vi "rsscope_core_global.vi"() -> ()   [LabVIEW 2014] (continued)
"Supported Models"="", "Instrument Options"="", "Flags"=0, "Help"="Return the statistic results of the specified measurement. If no parameter is specified, the result of the main measurement is returned. The main measurement is defined using RSSCOPE_ATTR_AMPT_MAIN_MEASUREMENT, RSSCOPE_ATTR_EYE_MAIN_MEASUREMENT, RSSCOPE_ATTR_HISTOGRAM_MAIN_MEASUREMENT, RSSCOPE_ATTR_JITTER_MAIN_MEASUREMENT, or RSSCOPE_ATTR_SPECTRUM_MAIN_MEASUREMENT.\n\nAvailable Repeated Capabilities:\nMeasurement: Meas1, Meas2, Meas3, Meas4, Meas5, Meas6, Meas7, Meas8, Meas9, Meas10\r\n\nRemote-control command(s):\nMEASurement<m>:RESult[:ACTual]?"}, {"Level"=3, "Class Only"=FALSE, "Identifier"="RSSCOPE_ATTR_READ_MAIN_MEASUREMENT_AVERAGE", "Descriptive Name"="Read Main Measurement Average", "Data Type"=1, "Command"="MEAS{Measurement}:RES:AVG?", "Access"=0, "Range Table"="", "Read Callback"="", "Write Callback"="", "Supported Models"="", "Instrument Options"="", "Flags"=0, "Help"="Return the statistic results of the specified measurement. If no parameter is specified, the result of the main measurement is returned. The main measurement is defined using RSSCOPE_ATTR_AMPT_MAIN_MEASUREMENT, RSSCOPE_ATTR_EYE_MAIN_MEASUREMENT, RSSCOPE_ATTR_HISTOGRAM_MAIN_MEASUREMENT, RSSCOPE_ATTR_JITTER_MAIN_MEASUREMENT, or RSSCOPE_ATTR_SPECTRUM_MAIN_MEASUREMENT.\n\nAvailable Repeated Capabilities:\nMeasurement: Meas1, Meas2, Meas3, Meas4, Meas5, Meas6, Meas7, Meas8, Meas9, Meas10\r\n\nRemote-control command(s):\nMEASurement<m>:RESult:AVG?"}, {"Level"=3, "Class Only"=FALSE, "Identifier"="RSSCOPE_ATTR_READ_MAIN_MEASUREMENT_EVENT_COUNT", "Descriptive Name"="Read Main Measurement Event Count", "Data Type"=1, "Command"="MEAS{Measurement}:RES:EVTC?", "Access"=0, "Range Table"="", "Read Callback"="", "Write Callback"="", "Supported Models"="", "Instrument Options"="", "Flags"=0, "Help"="Return the statistic results of the specified measurement. If no parameter is specified, the result of the main measurement is returned. The main measurement is defined using RSSCOPE_ATTR_AMPT_MAIN_MEASUREMENT, RSSCOPE_ATTR_EYE_MAIN_MEASUREMENT, RSSCOPE_ATTR_HISTOGRAM_MAIN_MEASUREMENT, RSSCOPE_ATTR_JITTER_MAIN_MEASUREMENT, or RSSCOPE_ATTR_SPECTRUM_MAIN_MEASUREMENT.\n\nAvailable Repeated Capabilities:\nMeasurement: Meas1, Meas2, Meas3, Meas4, Meas5, Meas6, Meas7, Meas8, Meas9, Meas10\r\n\nRemote-control command(s):\nMEASurement<m>:RESult:EVTCount?"}, {"Level"=3, "Class Only"=FALSE, "Identifier"="RSSCOPE_ATTR_READ_MAIN_MEASUREMENT_NEGATIVE_PEAK", "Descriptive Name"="Read Main Measurement Negative Peak", "Data Type"=1, "Command"="MEAS{Measurement}:RES:NPE?", "Access"=0, "Range Table"="", "Read Callback"="", "Write Callback"="", "Supported Models"="", "Instrument Options"="", "Flags"=0, "Help"="Return the statistic results of the specified measurement. If no parameter is specified, the result of the main measurement is returned. The main measurement is defined using RSSCOPE_ATTR_AMPT_MAIN_MEASUREMENT, RSSCOPE_ATTR_EYE_MAIN_MEASUREMENT, RSSCOPE_ATTR_HISTOGRAM_MAIN_MEASUREMENT, RSSCOPE_ATTR_JITTER_MAIN_MEASUREMENT, or RSSCOPE_ATTR_SPECTRUM_MAIN_MEASUREMENT.\n\nAvailable Repeated Capabilities:\nMeasurement: Meas1, Meas2, Meas3, Meas4, Meas5, Meas6, Meas7, Meas8, Meas9, Meas10\r\n\nRemote-control command(s):\nMEASurement<m>:RESult:NPEak?"}, {"Level"=3, "Class Only"=FALSE, "Identifier"="RSSCOPE_ATTR_READ_MAIN_MEASUREMENT_POSITIVE_PEAK", "Descriptive Name"="Read Main Measurement Positive Peak", "Data Type"=1, "Command"="MEAS{Measurement}:RES:PPE?", "Access"=0, "Range Table"="", "Read Callback"="", "Write Callback"="", "Supported Models"="", "Instrument Options"="", "Flags"=0, "Help"="Return the statistic results of the specified measurement. If no parameter is specified, the result of the main measurement is returned. The main measurement is defined using RSSCOPE_ATTR_AMPT_MAIN_MEASUREMENT, RSSCOPE_ATTR_EYE_MAIN_MEASUREMENT, RSSCOPE_ATTR_HISTOGRAM_MAIN_MEASUREMENT, RSSCOPE_ATTR_JITTER_MAIN_MEASUREMENT, or RSSCOPE_ATTR_SPECTRUM_MAIN_MEASUREMENT.\n\nAvailable Repeated Capabilities:\nMeasurement: Meas1, Meas2, Meas3, Meas4, Meas5, Meas6, Meas7, Meas8, Meas9, Meas10\r\n\nRemote-control command(s):\nMEASurement<m>:RESult:PPEak?"}, {"Level"=3, "Class Only"=FALSE, "Identifier"="RSSCOPE_ATTR_READ_MAIN_MEASUREMENT_RELIABILITY", "Descriptive Name"="Read Main Measurement Reliability", "Data Type"=1, "Command"="MEAS{Measurement}:RES:REL?", "Access"=0, "Range Table"="", "Read Callback"="", "Write Callback"="", "Supported Models"="", "Instrument Options"="", "Flags"=0, "Help"="Return the statistic results of the specified measurement. If no parameter is specified, the result of the main measurement is returned. The main measurement is defined using RSSCOPE_ATTR_AMPT_MAIN_MEASUREMENT, RSSCOPE_ATTR_EYE_MAIN_MEASUREMENT, RSSCOPE_ATTR_HISTOGRAM_MAIN_MEASUREMENT, RSSCOPE_ATTR_JITTER_MAIN_MEASUREMENT, or RSSCOPE_ATTR_SPECTRUM_MAIN_MEASUREMENT.\n\nAvailable Repeated Capabilities:\nMeasurement: Meas1, Meas2, Meas3, Meas4, Meas5, Meas6, Meas7, Meas8, Meas9, Meas10\r\n\nRemote-control command(s):\nMEASurement<m>:RESult:RELiability?"}, {"Level"=3, "Class Only"=FALSE, "Identifier"="RSSCOPE_ATTR_READ_MAIN_MEASUREMENT_RMS", "Descriptive Name"="Read Main Measurement RMS", "Data Type"=1, "Command"="MEAS{Measurement}:RES:RMS?", "Access"=0, "Range Table"="", "Read Callback"="", "Write Callback"="", "Supported Models"="", "Instrument Options"="", "Flags"=0, "Help"="Return the statistic results of the specified measurement. If no parameter is specified, the result of the main measurement is returned. The main measurement is defined using RSSCOPE_ATTR_AMPT_MAIN_MEASUREMENT, RSSCOPE_ATTR_EYE_MAIN_MEASUREMENT, RSSCOPE_ATTR_HISTOGRAM_MAIN_MEASUREMENT, RSSCOPE_ATTR_JITTER_MAIN_MEASUREMENT, or RSSCOPE_ATTR_SPECTRUM_MAIN_MEASUREMENT.\n\nAvailable Repeated Capabilities:\nMeasurement: Meas1, Meas2, Meas3, Meas4, Meas5, Meas6, Meas7, Meas8, Meas9, Meas10\r\n\nRemote-control command(s):\nMEASurement<m>:RESult:RMS?"}, {"Level"=3, "Class Only"=FALSE, "Identifier"="RSSCOPE_ATTR_READ_MAIN_MEASUREMENT_WAVEFORM_COUNT", "Descriptive Name"="Read Main Measurement Waveform Count", "Data Type"=1, "Command"="MEAS{Measurement}:RES:WFMC?", "Access"=0, "Range Table"="", "Read Callback"="", "Write Callback"="", "Supported Models"="", "Instrument Options"="", "Flags"=0, "Help"="Return the statistic results of the specified measurement. If no parameter is specified, the result of the main measurement is returned. The main measurement is defined using RSSCOPE_ATTR_AMPT_MAIN_MEASUREMENT, RSSCOPE_ATTR_EYE_MAIN_MEASUREMENT, RSSCOPE_ATTR_HISTOGRAM_MAIN_MEASUREMENT, RSSCOPE_ATTR_JITTER_MAIN_MEASUREMENT, or RSSCOPE_ATTR_SPECTRUM_MAIN_MEASUREMENT.\n\nAvailable Repeated Capabilities:\nMeasurement: Meas1, Meas2, Meas3, Meas4, Meas5, Meas6, Meas7, Meas8, Meas9, Meas10\r\n\nRemote-control command(s):\nMEASurement<m>:RESult:WFMCount?"}, {"Level"=3, "Class Only"=FALSE, "Identifier"="RSSCOPE_ATTR_READ_MAIN_MEASUREMENT_STANDARD_DEVIATION", "Descriptive Name"="Read Main Measurement Standard Deviation", "Data Type"=1, "Command"="MEAS{Measurement}:RES:STDD?", "Access"=0, "Range Table"="", "Read Callback"="", "Write Callback"="", "Supported Models"="", "Instrument Options"="", "Flags"=0, "Help"="Return the statistic results of the specified measurement. If no parameter is specified, the result of the main measurement is returned. The main measurement is defined using RSSCOPE_ATTR_AMPT_MAIN_MEASUREMENT, RSSCOPE_ATTR_EYE_MAIN_MEASUREMENT, RSSCOPE_ATTR_HISTOGRAM_MAIN_MEASUREMENT, RSSCOPE_ATTR_JITTER_MAIN_MEASUREMENT, or RSSCOPE_ATTR_SPECTRUM_MAIN_MEASUREMENT.\n\nAvailable Repeated Capabilities:\nMeasurement: Meas1, Meas2, Meas3, Meas4, Meas5, Meas6, Meas7, Meas8, Meas9, Meas10\r\n\nRemote-control command(s):\nMEASurement<m>:RESult:STDDev?"}, {"Level"=3, "Class Only"=FALSE, "Identifier"="RSSCOPE_ATTR_READ_REFERENCE_LEVEL_TOP_OUTER", "Descriptive Name"="Read Reference Level Top Outer", "Data Type"=1, "Command"="MEAS{Measurement}:REFL:RES:TOUT?", "Access"=0, "Range Table"="", "Read Callback"="", "Write Callback"="", "Supported Models"="", "Instrument Options"="", "Flags"=0, "Help"="Returns the area above the high signal level which is still considered to be high level.\n\nAvailable Repeated Capabilities:\nMeasurement: Meas1, Meas2, Meas3, Meas4, Meas5, Meas6, Meas7, Meas8, Meas9, Meas10\r\n\nRemote-control command(s):\nMEASurement<m>:REFLevel:RESult:TOUTer?"}, {"Level"=3, "Class Only"=FALSE, "Identifier"="RSSCOPE_ATTR_READ_REFERENCE_LEVEL_TOP_INNER", "Descriptive Name"="Read Reference Level Top Inner", "Data Type"=1, "Command"="MEAS{Measurement}:REFL:RES:TINN?", "Access"=0, "Range Table"="", "Read Callback"="", "Write Callback"="", "Supported Models"="", "Instrument Options"="", "Flags"=0, "Help"="Returns the area beneath the high signal level which is still considered to be high level.\n\nAvailable Repeated Capabilities:\nMeasurement: Meas1, Meas2, Meas3, Meas4, Meas5, Meas6, Meas7, Meas8, Meas9, Meas10\r\n\nRemote-control command(s):\nMEASurement<m>:REFLevel:RESult:TINNer?"}, {"Level"=3, "Class Only"=FALSE, "Identifier"="RSSCOPE_ATTR_READ_REFERENCE_LEVEL_BOTTOM_INNER", "Descriptive Name"="Read Reference Level Bottom Inner", "Data Type"=1, "Command"="MEAS{Measurement}:REFL:RES:BINN?", "Access"=0, "Range Table"="", "Read Callback"="", "Write Callback"="", "Supported Models"="", "Instrument Options"="", "Flags"=0, "Help"="Returns the area above the low signal level which is still considered to be low level.\n\nAvailable Repeated Capabilities:\nMeasurement: Meas1, Meas2, Meas3, Meas4, Meas5, Meas6, Meas7, Meas8, Meas9, Meas10\r\n\nRemote-control command(s):\nMEASurement<m>:REFLevel:RESult:BINNer?"}, {"Level"=3, "Class Only"=FALSE, "Identifier"="RSSCOPE_ATTR_READ_REFERENCE_LEVEL_BOTTOM_OUTER", "Descriptive Name"="Read Reference Level Bottom Outer", "Data Type"=1, "Command"="MEAS{Measurement}:REFL:RES:BOUT?", "Access"=0, "Range Table"="", "Read Callback"="", "Write Callback"="", "Supported Models"="", "Instrument Options"="", "Flags"=0, "Help"="Defines an area beneath the low signal level which is still considered to be low level.\n\nAvailable Repeated Capabilities:\nMeasurement: Meas1, Meas2, Meas3, Meas4, Meas5, Meas6, Meas7, Meas8, Meas9, Meas10\r\n\nRemote-control command(s):\nMEASurement<m>:REFLevel:RESult:BOUTer?"}, {"Level"=3, "Class Only"=FALSE, "Identifier"="RSSCOPE_ATTR_READ_REFERENCE_LEVEL_LOWER", "Descriptive Name"="Read Reference Level Lower", "Data Type"=1, "Command"="MEAS{Measurement}:REFL:RES:LOW?", "Access"=0, "Range Table"="", "Read Callback"="", "Write Callback"="", "Supported Models"="", "Instrument Options"="", "Flags"=0, "Help"="Return the lower reference level.\n\nAvailable Repeated Capabilities:\nMeasurement: Meas1, Meas2, Meas3, Meas4, Meas5, Meas6, Meas7, Meas8, Meas9, Meas10\r\n\nRemote-control command(s):\nMEASurement<m>:REFLevel:RESult:LOWer?"}, {"Level"=3, "Class Only"=FALSE, "Identifier"="RSSCOPE_ATTR_READ_REFERENCE_LEVEL_MIDDLE", "Descriptive Name"="Read Reference Level Middle", "Data Type"=1, "Command"="MEAS{Measurement}:REFL:RES:MIDD?", "Access"=0, "Range Table"="", "Read Callback"="", "Write Callback"="", "Supported Models"="", "Instrument Options"="", "Flags"=0, "Help"="Return the middle reference level.\n\nAvailable Repeated Capabilities:\nMeasurement: Meas1, Meas2, Meas3, Meas4, Meas5, Meas6, Meas7, Meas8, Meas9, Meas10\r\n\nRemote-control command(s):\nMEASurement<m>:REFLevel:RESult:MIDDle?"}, {"Level"=3, "Class Only"=FALSE, "Identifier"="RSSCOPE_ATTR_READ_REFERENCE_LEVEL_UPPER", "Descriptive Name"="Read Reference Level Upper", "Data Type"=1, "Command"="MEAS{Measurement}:REFL:RES:UPP?", "Access"=0, "Range Table"="", "Read Callback"="", "Write Callback"="", "Supported Models"="", "Instrument Options"="", "Flags"=0, "Help"="Return the upper reference level.\n\nAvailable Repeated Capabilities:\nMeasurement: Meas1, Meas2, Meas3, Meas4, Meas5, Meas6, Meas7, Meas8, Meas9, Meas10\r\n\nRemote-control command(s):\nMEASurement<m>:REFLevel:RESult:UPPer?"}, {"Level"=3, "Class Only"=FALSE, "Identifier"="RSSCOPE_ATTR_READ_REFERENCE_LEVEL_SIGNAL_LOW", "Descriptive Name"="Read Reference Level Signal Low", "Data Type"=1, "Command"="MEAS{Measurement}:REFL:RES:SIGL?", "Access"=0, "Range Table"="", "Read Callback"="", "Write Callback"="", "Supported Models"="", "Instrument Options"="", "Flags"=0, "Help"="Return the signal value that represents a low level.\n\nAvailable Repeated Capabilities:\nMeasurement: Meas1, Meas2, Meas3, Meas4, Meas5, Meas6, Meas7, Meas8, Meas9, Meas10\r\n\nRemote-control command(s):\nMEASurement<m>:REFLevel:RESult:SIGLow?"}, {"Level"=3, "Class Only"=FALSE, "Identifier"="RSSCOPE_ATTR_READ_REFERENCE_LEVEL_SIGNAL_HIGH", "Descriptive Name"="Read Reference Level Signal High", "Data Type"=1, "Command"="MEAS{Measurement}:REFL:RES:SIGH?", "Access"=0, "Range Table"="", "Read Callback"="", "Write Callback"="", "Supported Models"="", "Instrument Options"="", "Flags"=0, "Help"="Return the signal value that represents a high level.\n\nAvailable Repeated Capabilities:\nMeasurement: Meas1, Meas2, Meas3, Meas4, Meas5, Meas6, Meas7, Meas8, Meas9, Meas10\r\n\nRemote-control command(s):\nMEASurement<m>:REFLevel:RESult:SIGHigh?"}, {"Level"=3, "Class Only"=FALSE, "Identifier"="RSSCOPE_ATTR_SPECTRUM_MEASUREMENT_HARMONICS_RESULTS_NUMBER", "Descriptive Name"="Spectrum Measurement Harmonics Results Number", "Data Type"=0, "Command"="MEAS{Measurement}:RES:COUN? HAR", "Access"=0, "Range Table"="", "Read Callback"="", "Write Callback"="", "Supported Models"="", "Instrument Options"="", "Flags"=0, "Help"="Returns the number of result groups that are returned by harmonics search.\n\nAvailable Repeated Capabilities:\nMeasurement: Meas1, Meas2, Meas3, Meas4, Meas5, Meas6, Meas7, Meas8, Meas9, Meas10\r\n\nRemote-control command(s):\nMEASurement<m>:RESult:COUNt? HAR"}, {"Level"=3, "Class Only"=FALSE, "Identifier"="RSSCOPE_ATTR_DISPLAY_RESULT_LINES", "Descriptive Name"="Display Result Lines", "Data Type"=3, "Command"="MEAS{Measurement}:DISP:RES", "Access"=2, "Range Table"="", "Read Callback"="", "Write Callback"="", "Supported Models"="", "Instrument Options"="", "Flags"=0, "Help"="If enabled, the intermediate result lines required to obtain the measurement result (e.g. signal thresholds) are displayed in the measurement diagram.\n\nAvailable Repeated Capabilities:\nMeasurement: Meas1, Meas2, Meas3, Meas4, Meas5, Meas6, Meas7, Meas8, Meas9, Meas10\r\n\nRemote-control command(s):\nMEASurement<m>:DISPlay:RESults"}, {"Level"=3, "Class Only"=FALSE, "Identifier"="RSSCOPE_ATTR_DISPLAY_REFERENCE_LEVELS", "Descriptive Name"="Display Reference Levels", "Data Type"=3, "Command"="MEAS{Measurement}:DISP:LEV", "Access"=2, "Range Table"="", "Read Callback"="", "Write Callback"="", "Supported Models"="", "Instrument Options"="", "Flags"=0, "Help"="If enabled, the reference levels used for the measurement are displayed in the diagram.\n\nAvailable Repeated Capabilities:\nMeasurement: Meas1, Meas2, Meas3, Meas4, Meas5, Meas6, Meas7, Meas8, Meas9, Meas10\r\n\nRemote-control command(s):\nMEASurement<m>:DISPlay:LEVels"}, {"Level"=3, "Class Only"=FALSE, "Identifier"="RSSCOPE_ATTR_DISPLAY_RESULT_TABLE_DEFAULT_POSITION", "Descriptive Name"="Display Result Table Default Position", "Data Type"=0, "Command"="DISP:RES:MEP", "Access"=2, "Range Table"="RsScope_rngDisplayResultTableDefaultPosition", "Read Callback"="", "Write Callback"="", "Supported Models"="", "Instrument Options"="", "Flags"=0, "Help"="Defines the position of the measurement results on the display.\n\nAvailable Repeated Capabilities:\nNone\n\nRemote-control command(s):\nDISPlay:RESultboxes:MEPosition"}, {"Level"=3, "Class Only"=FALSE, "Identifier"="RSSCOPE_ATTR_DISPLAY_GROUP_RESULT_DIALOGS", "Descriptive Name"="Display Group Result Dialogs", "Data Type"=3, "Command"="MEAS:DISP:GRO", "Access"=2, "Range Table"="", "Read Callback"="", "Write Callback"="", "Supported Models"="", "Instrument Options"="", "Flags"=0, "Help"="If ON, all measurement results are shown in one result box. If disabled, the results of each measurement group are shown in a separate result box. The default position is ignored.\n\nAvailable Repeated Capabilities:\nNone\n\nRemote-control command(s):\nMEASurement<m>:DISPlay:GROuping"}, {"Level"=3, "Class Only"=TRUE, "Identifier"="", "Descriptive Name"="Raw", "Data Type"=0, "Command"="", "Access"=0, "Range Table"="", "Read Callback"="", "Write Callback"="", "Supported Models"="", "Instrument Options"="", "Flags"=0, "Help"="Use members in this class to retrieve the raw text returned by the instrument for low-level main measurements."}, {"Level"=4, "Class Only"=FALSE, "Identifier"="RSSCOPE_ATTR_READ_MAIN_MEASUREMENT_ACTUAL_STRING", "Descriptive Name"="Read Main Measurement Actual String", "Data Type"=2, "Command"="MEAS{Measurement}:RES?", "Access"=0, "Range Table"="", "Read Callback"="", "Write Callback"="", "Supported Models"="", "Instrument Options"="", "Flags"=0, "Help"="Return the statistic results of the specified measurement. If no parameter is specified, the result of the main measurement is returned. The main measurement is defined using RSSCOPE_ATTR_AMPT_MAIN_MEASUREMENT, RSSCOPE_ATTR_EYE_MAIN_MEASUREMENT, RSSCOPE_ATTR_HISTOGRAM_MAIN_MEASUREMENT, RSSCOPE_ATTR_JITTER_MAIN_MEASUREMENT, or RSSCOPE_ATTR_SPECTRUM_MAIN_MEASUREMENT.\n\nAvailable Repeated Capabilities:\nMeasurement: Meas1, Meas2, Meas3, Meas4, Meas5, Meas6, Meas7, Meas8, Meas9, Meas10\r\n\nRemote-control command(s):\nMEASurement<m>:RESult[:ACTual]?"}, {"Level"=4, "Class Only"=FALSE, "Identifier"="RSSCOPE_ATTR_READ_MAIN_MEASUREMENT_AVERAGE_STRING", "Descriptive Name"="Read Main Measurement Average String", "Data Type"=2, "Command"="MEAS{Measurement}:RES:AVG?", "Access"=0, "Range Table"="", "Read Callback"="", "Write Callback"="", "Supported Models"="", "Instrument Options"="", "Flags"=0, "Help"="Return the statistic results of the specified measurement. If no parameter is specified, the result of the main measurement is returned. The main measurement is defined using RSSCOPE_ATTR_AMPT_MAIN_MEASUREMENT, RSSCOPE_ATTR_EYE_MAIN_MEASUREMENT, RSSCOPE_ATTR_HISTOGRAM_MAIN_MEASUREMENT, RSSCOPE_ATTR_JITTER_MAIN_MEASUREMENT, or RSSCOPE_ATTR_SPECTRUM_MAIN_MEASUREMENT.\n\nAvailable Repeated Capabilities:\nMeasurement: Meas1, Meas2, Meas3, Meas4, Meas5, Meas6, Meas7, Meas8, Meas9, Meas10\r\n\nRemote-control command(s):\nMEASurement<m>:RESult:AVG?"}, {"Level"=4, "Class Only"=FALSE, "Identifier"="RSSCOPE_ATTR_READ_MAIN_MEASUREMENT_EVENT_COUNT_STRING", "Descriptive Name"="Read Main Measurement Event Count String", "Data Type"=2, "Command"="MEAS{Measurement}:RES:EVTC?", "Access"=0, "Range Table"="", "Read Callback"="", "Write Callback"="", "Supported Models"="", "Instrument Options"="", "Flags"=0, "Help"="Return the statistic results of the specified measurement. If no parameter is specified, the result of the main measurement is returned. The main measurement is defined using RSSCOPE_ATTR_AMPT_MAIN_MEASUREMENT, RSSCOPE_ATTR_EYE_MAIN_MEASUREMENT, RSSCOPE_ATTR_HISTOGRAM_MAIN_MEASUREMENT, RSSCOPE_ATTR_JITTER_MAIN_MEASUREMENT, or RSSCOPE_ATTR_SPECTRUM_MAIN_MEASUREMENT.\n\nAvailable Repeated Capabilities:\nMeasurement: Meas1, Meas2, Meas3, Meas4, Meas5, Meas6, Meas7, Meas8, Meas9, Meas10\r\n\nRemote-control command(s):\nMEASurement<m>:RESult:EVTCount?"}, {"Level"=4, "Class Only"=FALSE, "Identifier"="RSSCOPE_ATTR_READ_MAIN_MEASUREMENT_NEGATIVE_PEAK_STRING", "Descriptive Name"="Read Main Measurement Negative Peak String", "Data Type"=2, "Command"="MEAS{Measurement}:RES:NPE?", "Access"=0, "Range Table"="", "Read Callback"="", "Write Callback"="", "Supported Models"="", "Instrument Options"="", "Flags"=0, "Help"="Return the statistic results of the specified measurement. If no parameter is specified, the result of the main measurement is returned. The main measurement is defined using RSSCOPE_ATTR_AMPT_MAIN_MEASUREMENT, RSSCOPE_ATTR_EYE_MAIN_MEASUREMENT, RSSCOPE_ATTR_HISTOGRAM_MAIN_MEASUREMENT, RSSCOPE_ATTR_JITTER_MAIN_MEASUREMENT, or RSSCOPE_ATTR_SPECTRUM_MAIN_MEASUREMENT.\n\nAvailable Repeated Capabilities:\nMeasurement: Meas1, Meas2, Meas3, Meas4, Meas5, Meas6, Meas7, Meas8, Meas9, Meas10\r\n\nRemote-control command(s):\nMEASurement<m>:RESult:NPEak?"}, {"Level"=4, "Class Only"=FALSE, "Identifier"="RSSCOPE_ATTR_READ_MAIN_MEASUREMENT_POSITIVE_PEAK_STRING", "Descriptive Name"="Read Main Measurement Positive Peak String", "Data Type"=2, "Command"="MEAS{Measurement}:RES:PPE?", "Access"=0, "Range Table"="", "Read Callback"="", "Write Callback"="", "Supported Models"="", "Instrument Options"="", "Flags"=0, "Help"="Return the statistic results of the specified measurement. If no parameter is specified, the result of the main measurement is returned. The main measurement is defined using RSSCOPE_ATTR_AMPT_MAIN_MEASUREMENT, RSSCOPE_ATTR_EYE_MAIN_MEASUREMENT, RSSCOPE_ATTR_HISTOGRAM_MAIN_MEASUREMENT, RSSCOPE_ATTR_JITTER_MAIN_MEASUREMENT, or RSSCOPE_ATTR_SPECTRUM_MAIN_MEASUREMENT.\n\nAvailable Repeated Capabilities:\nMeasurement: Meas1, Meas2, Meas3, Meas4, Meas5, Meas6, Meas7, Meas8, Meas9, Meas10\r\n\nRemote-control command(s):\nMEASurement<m>:RESult:PPEak?"}, {"Level"=4, "Class Only"=FALSE, "Identifier"="RSSCOPE_ATTR_READ_MAIN_MEASUREMENT_RELIABILITY_STRING", "Descriptive Name"="Read Main Measurement Reliability String", "Data Type"=2, "Command"="MEAS{Measurement}:RES:REL?", "Access"=0, "Range Table"="", "Read Callback"="", "Write Callback"="", "Supported Models"="", "Instrument Options"="", "Flags"=0, "Help"="Return the statistic results of the specified measurement. If no parameter is specified, the result of the main measurement is returned. The main measurement is defined using RSSCOPE_ATTR_AMPT_MAIN_MEASUREMENT, RSSCOPE_ATTR_EYE_MAIN_MEASUREMENT, RSSCOPE_ATTR_HISTOGRAM_MAIN_MEASUREMENT, RSSCOPE_ATTR_JITTER_MAIN_MEASUREMENT, or RSSCOPE_ATTR_SPECTRUM_MAIN_MEASUREMENT.\n\nAvailable Repeated Capabilities:\nMeasurement: Meas1, Meas2, Meas3, Meas4, Meas5, Meas6, Meas7, Meas8, Meas9, Meas10\r\n\nRemote-control command(s):\nMEASurement<m>:RESult:RELiability?"}, {"Level"=4, "Class Only"=FALSE, "Identifier"="RSSCOPE_ATTR_READ_MAIN_MEASUREMENT_RMS_STRING", "Descriptive Name"="Read Main Measurement RMS String", "Data Type"=2, "Command"="MEAS{Measurement}:RES:RMS?", "Access"=0, "Range Table"="", "Read Callback"="", "Write Callback"="", "Supported Models"="", "Instrument Options"="", "Flags"=0, "Help"="Return the statistic results of the specified measurement. If no parameter is specified, the result of the main measurement is returned. The main measurement is defined using RSSCOPE_ATTR_AMPT_MAIN_MEASUREMENT, RSSCOPE_ATTR_EYE_MAIN_MEASUREMENT, RSSCOPE_ATTR_HISTOGRAM_MAIN_MEASUREMENT, RSSCOPE_ATTR_JITTER_MAIN_MEASUREMENT, or RSSCOPE_ATTR_SPECTRUM_MAIN_MEASUREMENT.\n\nAvailable Repeated Capabilities:\nMeasurement: Meas1, Meas2, Meas3, Meas4, Meas5, Meas6, Meas7, Meas8, Meas9, Meas10\r\n\nRemote-control command(s):\nMEASurement<m>:RESult:RMS?"}, {"Level"=4, "Class Only"=FALSE, "Identifier"="RSSCOPE_ATTR_READ_MAIN_MEASUREMENT_WAVEFORM_COUNT_STRING", "Descriptive Name"="Read Main Measurement Waveform Count String", "Data Type"=2, "Command"="MEAS{Measurement}:RES:WFMC?", "Access"=0, "Range Table"="", "Read Callback"="", "Write Callback"="", "Supported Models"="", "Instrument Options"="", "Flags"=0, "Help"="Return the statistic results of the specified measurement. If no parameter is specified, the result of the main measurement is returned. The main measurement is defined using RSSCOPE_ATTR_AMPT_MAIN_MEASUREMENT, RSSCOPE_ATTR_EYE_MAIN_MEASUREMENT, RSSCOPE_ATTR_HISTOGRAM_MAIN_MEASUREMENT, RSSCOPE_ATTR_JITTER_MAIN_MEASUREMENT, or RSSCOPE_ATTR_SPECTRUM_MAIN_MEASUREMENT.\n\nAvailable Repeated Capabilities:\nMeasurement: Meas1, Meas2, Meas3, Meas4, Meas5, Meas6, Meas7, Meas8, Meas9, Meas10\r\n\nRemote-control command(s):\nMEASurement<m>:RESult:WFMCount?"}, {"Level"=4, "Class Only"=FALSE, "Identifier"="RSSCOPE_ATTR_READ_MAIN_MEASUREMENT_STANDARD_DEVIATION_STRING", "Descriptive Name"="Read Main Measurement Standard Deviation String", "Data Type"=2, "Command"="MEAS{Measurement}:RES:STDD?", "Access"=0, "Range Table"="", "Read Callback"="", "Write Callback"="", "Supported Models"="", "Instrument Options"="", "Flags"=0, "Help"="Return the statistic results of the specified measurement. If no parameter is specified, the result of the main measurement is returned. The main measurement is defined using RSSCOPE_ATTR_AMPT_MAIN_MEASUREMENT, RSSCOPE_ATTR_EYE_MAIN_MEASUREMENT, RSSCOPE_ATTR_HISTOGRAM_MAIN_MEASUREMENT, RSSCOPE_ATTR_JITTER_MAIN_MEASUREMENT, or RSSCOPE_ATTR_SPECTRUM_MAIN_MEASUREMENT.\n\nAvailable Repeated Capabilities:\nMeasurement: Meas1, Meas2, Meas3, Meas4, Meas5, Meas6, Meas7, Meas8, Meas9, Meas10\r\n\nRemote-control command(s):\nMEASurement<m>:RESult:STDDev?"}, {"Level"=1, "Class Only"=TRUE, "Identifier"="", "Descriptive Name"="Reference Level", "Data Type"=0, "Command"="", "Access"=0, "Range Table"="", "Read Callback"="", "Write Callback"="", "Supported Models"="", "Instrument Options"="", "Flags"=0, "Help"="Contains Reference Level configuration."}, {"Level"=2, "Class Only"=FALSE, "Identifier"="RSSCOPE_ATTR_REFERENCE_LEVEL_MODE", "Descriptive Name"="Reference Level Mode", "Data Type"=0, "Command"="REFL{WfmSuffix}:LDET", "Access"=2, "Range Table"="rsscope_rngAutoManual", "Read Callback"="", "Write Callback"="", "Supported Models"="", "Instrument Options"="", "Flags"=0, "Help"="Defines whether the reference level is configured manually or automatically.\n\nAvailable Repeated Capabilities:\nWfmSuffix: WfmNone, WfmC1W1, WfmC1W2, WfmC1W3, WfmC2W1, WfmC2W2, WfmC2W3, WfmC3W1, WfmC3W2, WfmC3W3, WfmC4W1, WfmC4W2, WfmC4W3, WfmMath1, WfmMath2, WfmMath3, WfmMath4, WfmRef1, WfmRef2, WfmRef3, WfmRef4, WfmXY1, WfmXY2, WfmXY3, WfmXY4, WfmMeas1, WfmMeas2, WfmMeas3, WfmMeas4, WfmMeas5, WfmMeas6, WfmMeas7, WfmMeas8, WfmSbus1, WfmSbus2, WfmSbus3, WfmSbus4, WfmD0, WfmD1, WfmD2, WfmD3, WfmD4, WfmD5, WfmD6, WfmD7, WfmD8, WfmD9, WfmD10, WfmD11, WfmD12, WfmD13, WfmD14, WfmD15, WfmMSO1, WfmMSO2, WfmMSO3, WfmMSO4, WfmTRK1, WfmTRK2, WfmTRK3, WfmTRK4, WfmTRK5, WfmTRK6, WfmTRK7, WfmTRK8, WfmSpectrum1, WfmSpectrum2, WfmSpectrum3, WfmSpectrum4, WfmSG1TL1, WfmSG1TL2, WfmSG2TL1, WfmSG2TL2, WfmSG3TL1, WfmSG3TL2, WfmSG4TL1, WfmSG4TL2, WfmEye1, WfmEye2, WfmEye3, WfmEye4, WfmZ1V1, WfmZ1V2, WfmZ1V3, WfmZ1V4, WfmZ1I1, WfmZ1I2, WfmZ1I3, WfmZ1I4, WfmZ2V1, WfmZ2V2, WfmZ2V3, WfmZ2V4, WfmZ2I1, WfmZ2I2, WfmZ2I3, WfmZ2I4, WfmDiff1, WfmDiff2, WfmCommon1, WfmCommon2, WfmTDRZ, WfmTDRH, WfmTDRR, WfmMath5, WfmMath6, WfmMath7, WfmMath8, WfmSpectrum5, WfmSpectrum6, WfmSpectrum7, WfmSpectrum8, WfmSG5TL1, WfmSG5TL2, WfmSG6TL1, WfmSG6TL2, WfmSG7TL1, WfmSG7TL2, WfmSG8TL1, WfmSG8TL2, WfmHP1, WfmHP2, WfmHP3, WfmHP4, WfmHP5, WfmHP6, WfmHP7, WfmHP8, WfmHP9, WfmHP10, WfmBathtub1, WfmBathMeas1, WfmStepResp1, WfmSRHist1, WfmSDHist1, WfmTJHist1, WfmDJHist1, WfmDDJHist1, WfmPJHist1, WfmRJOHist1, WfmSRTrack1, WfmTJTrack1, WfmDJTrack1, WfmDDJTrack1, WfmPJTrack1, WfmRJTrack1, WfmTJSpectrum1, WfmDDJSpectrum1, WfmPJSpectrum1, WfmRJSpectrum1, WfmSEye1, WfmBathtub2, WfmBathMeas2, WfmStepResp2, WfmSRHist2, WfmSDHist2, WfmTJHist2, WfmDJHist2, WfmDDJHist2, WfmPJHist2, WfmRJOHist2, WfmSRTrack2, WfmSDTrack2, WfmTJTrack2, WfmDDJTrack2, WfmPJTrack2, WfmRJTrack2, WfmTJSpectrum2, WfmDDJSpectrum2, WfmPJSpectrum2, WfmRJSpectrum2, WfmSEye2, WfmNBathtub1, WfmNBathMeas1, WfmTNHist1, WfmDNHist1, WfmDDNHist1, WfmPNHist1, WfmRNOTrack1, WfmTNTrack1, WfmDDNTrack1, WfmPNTrack1, WfmRNTrack1, WfmTNSpectrum1, WfmDDNSpectrum1, WfmPNSpectrum1, WfmRNSpectrum1, WfmNBathtub2, WfmNBathMeas2, WfmTNHist2, WfmDNHist2, WfmDDNHist2, WfmPNHist2, WfmRNOHist2, WfmTNTrack2, WfmDDNTrack2, WfmPNTrack2, WfmRNTrack2, WfmTNSpectrum2, WfmDDNSpectrum2, WfmPNSpectrum2, WfmRNSpectrum2, WfmPJDHist1, WfmBUJHist1, WfmRJHist1, WfmPJDTrack1, WfmPJDSpectrum1, WfmPJDHist2, WfmBUJHist2, WfmRJHist2, WfmPJDTrack2, WfmPJDSpectrum2, WfmPNDHist1, WfmBUNHist1, WfmRNHist1, WfmPNDTrack1, WfmPNDSpectrum1, WfmPNDHist2, WfmBUNHist2, WfmRNHist2, WfmPNDTrack2, WfmPNDSpectrum2\r\n\nRemote-control command(s):\nREFLevel<m>:LDETection"}, {"Level"=2, "Class Only"=FALSE, "Identifier"="RSSCOPE_ATTR_REFERENCE_LEVEL_RELATIVE_LEVELS", "Descriptive Name"="Reference Level Relative Levels", "Data Type"=0, "Command"="REFL{WfmSuffix}:REL:MODE", "Access"=2, "Range Table"="rsscope_rngRefLevelRelative", "Read Callback"="", "Write Callback"="", "Supported Models"="", "Instrument Options"="", "Flags"=0, "Help"="The lower, middle and upper reference levels, defined as percentages of the high signal level.\n\nNote:\nFor user defined values set USER and use these attributes:\n\nRSSCOPE_ATTR_USER_REFERENCE_RELATIVE_LOWER_LEVEL\nRSSCOPE_ATTR_USER_REFERENCE_RELATIVE_MIDDLE_LEVEL\nRSSCOPE_ATTR_USER_REFERENCE_RELATIVE_UPPER_LEVEL\n\nAvailable Repeated Capabilities:\nWfmSuffix: WfmNone, WfmC1W1, WfmC1W2, WfmC1W3, WfmC2W1, WfmC2W2, WfmC2W3, WfmC3W1, WfmC3W2, WfmC3W3, WfmC4W1, WfmC4W2, WfmC4W3, WfmMath1, WfmMath2, WfmMath3, WfmMath4, WfmRef1, WfmRef2, WfmRef3, WfmRef4, WfmXY1, WfmXY2, WfmXY3, WfmXY4, WfmMeas1, WfmMeas2, WfmMeas3, WfmMeas4, WfmMeas5, WfmMeas6, WfmMeas7, WfmMeas8, WfmSbus1, WfmSbus2, WfmSbus3, WfmSbus4, WfmD0, WfmD1, WfmD2, WfmD3, WfmD4, WfmD5, WfmD6, WfmD7, WfmD8, WfmD9, WfmD10, WfmD11, WfmD12, WfmD13, WfmD14, WfmD15, WfmMSO1, WfmMSO2, WfmMSO3, WfmMSO4, WfmTRK1, WfmTRK2, WfmTRK3, WfmTRK4, WfmTRK5, WfmTRK6, WfmTRK7, WfmTRK8, WfmSpectrum1, WfmSpectrum2, WfmSpectrum3, WfmSpectrum4, WfmSG1TL1, WfmSG1TL2, WfmSG2TL1, WfmSG2TL2, WfmSG3TL1, WfmSG3TL2, WfmSG4TL1, WfmSG4TL2, WfmEye1, WfmEye2, WfmEye3, WfmEye4, WfmZ1V1, WfmZ1V2, WfmZ1V3, WfmZ1V4, WfmZ1I1, WfmZ1I2, WfmZ1I3, WfmZ1I4, WfmZ2V1, WfmZ2V2, WfmZ2V3, WfmZ2V4, WfmZ2I1, WfmZ2I2, WfmZ2I3, WfmZ2I4, WfmDiff1, WfmDiff2, WfmCommon1, WfmCommon2, WfmTDRZ, WfmTDRH, WfmTDRR, WfmMath5, WfmMath6, WfmMath7, WfmMath8, WfmSpectrum5, WfmSpectrum6, WfmSpectrum7, WfmSpectrum8, WfmSG5TL1, WfmSG5TL2, WfmSG6TL1, WfmSG6TL2, WfmSG7TL1, WfmSG7TL2, WfmSG8TL1, WfmSG8TL2, WfmHP1, WfmHP2, WfmHP3, WfmHP4, WfmHP5, WfmHP6, WfmHP7, WfmHP8, WfmHP9, WfmHP10, WfmBathtub1, WfmBathMeas1, WfmStepResp1, WfmSRHist1, WfmSDHist1, WfmTJHist1, WfmDJHist1, WfmDDJHist1, WfmPJHist1, WfmRJOHist1, WfmSRTrack1, WfmTJTrack1, WfmDJTrack1, WfmDDJTrack1, WfmPJTrack1, WfmRJTrack1, WfmTJSpectrum1, WfmDDJSpectrum1, WfmPJSpectrum1, WfmRJSpectrum1, WfmSEye1, WfmBathtub2, WfmBathMeas2, WfmStepResp2, WfmSRHist2, WfmSDHist2, WfmTJHist2, WfmDJHist2, WfmDDJHist2, WfmPJHist2, WfmRJOHist2, WfmSRTrack2, WfmSDTrack2, WfmTJTrack2, WfmDDJTrack2, WfmPJTrack2, WfmRJTrack2, WfmTJSpectrum2, WfmDDJSpectrum2, WfmPJSpectrum2, WfmRJSpectrum2, WfmSEye2, WfmNBathtub1, WfmNBathMeas1, WfmTNHist1, WfmDNHist1, WfmDDNHist1, WfmPNHist1, WfmRNOTrack1, WfmTNTrack1, WfmDDNTrack1, WfmPNTrack1, WfmRNTrack1, WfmTNSpectrum1, WfmDDNSpectrum1, WfmPNSpectrum1, WfmRNSpectrum1, WfmNBathtub2, WfmNBathMeas2, WfmTNHist2, WfmDNHist2, WfmDDNHist2, WfmPNHist2, WfmRNOHist2, WfmTNTrack2, WfmDDNTrack2, WfmPNTrack2, WfmRNTrack2, WfmTNSpectrum2, WfmDDNSpectrum2, WfmPNSpectrum2, WfmRNSpectrum2, WfmPJDHist1, WfmBUJHist1, WfmRJHist1, WfmPJDTrack1, WfmPJDSpectrum1, WfmPJDHist2, WfmBUJHist2, WfmRJHist2, WfmPJDTrack2, WfmPJDSpectrum2, WfmPNDHist1, WfmBUNHist1, WfmRNHist1, WfmPNDTrack1, WfmPNDSpectrum1, WfmPNDHist2, WfmBUNHist2, WfmRNHist2, WfmPNDTrack2, WfmPNDSpectrum2\r\n\nRemote-control command(s):\nREFLevel<m>:RELative:MODE"}, {"Level"=2, "Class Only"=FALSE, "Identifier"="RSSCOPE_ATTR_REFERENCE_LEVEL_USER_LEVEL", "Descriptive Name"="Reference Level User Level", "Data Type"=0, "Command"="REFL{WfmSuffix}:USRL", "Access"=2, "Range Table"="rsscope_rngUserLevel", "Read Callback"="", "Write Callback"="", "Supported Models"="", "Instrument Options"="", "Flags"=0, "Help"="Defines whether the user-defined signal levels or user-defined reference levels are used for the measurements.\n\nAvailable Repeated Capabilities:\nWfmSuffix: WfmNone, WfmC1W1, WfmC1W2, WfmC1W3, WfmC2W1, WfmC2W2, WfmC2W3, WfmC3W1, WfmC3W2, WfmC3W3, WfmC4W1, WfmC4W2, WfmC4W3, WfmMath1, WfmMath2, WfmMath3, WfmMath4, WfmRef1, WfmRef2, WfmRef3, WfmRef4, WfmXY1, WfmXY2, WfmXY3, WfmXY4, WfmMeas1, WfmMeas2, WfmMeas3, WfmMeas4, WfmMeas5, WfmMeas6, WfmMeas7, WfmMeas8, WfmSbus1, WfmSbus2, WfmSbus3, WfmSbus4, WfmD0, WfmD1, WfmD2, WfmD3, WfmD4, WfmD5, WfmD6, WfmD7, WfmD8, WfmD9, WfmD10, WfmD11, WfmD12, WfmD13, WfmD14, WfmD15, WfmMSO1, WfmMSO2, WfmMSO3, WfmMSO4, WfmTRK1, WfmTRK2, WfmTRK3, WfmTRK4, WfmTRK5, WfmTRK6, WfmTRK7, WfmTRK8, WfmSpectrum1, WfmSpectrum2, WfmSpectrum3, WfmSpectrum4, WfmSG1TL1, WfmSG1TL2, WfmSG2TL1, WfmSG2TL2, WfmSG3TL1, WfmSG3TL2, WfmSG4TL1, WfmSG4TL2, WfmEye1, WfmEye2, WfmEye3, WfmEye4, WfmZ1V1, WfmZ1V2, WfmZ1V3, WfmZ1V4, WfmZ1I1, WfmZ1I2, WfmZ1I3, WfmZ1I4, WfmZ2V1, WfmZ2V2, WfmZ2V3, WfmZ2V4, WfmZ2I1, WfmZ2I2, WfmZ2I3, WfmZ2I4, WfmDiff1, WfmDiff2, WfmCommon1, WfmCommon2, WfmTDRZ, WfmTDRH, WfmTDRR, WfmMath5, WfmMath6, WfmMath7, WfmMath8, WfmSpectrum5, WfmSpectrum6, WfmSpectrum7, WfmSpectrum8, WfmSG5TL1, WfmSG5TL2, WfmSG6TL1, WfmSG6TL2, WfmSG7TL1, WfmSG7TL2, WfmSG8TL1, WfmSG8TL2, WfmHP1, WfmHP2, WfmHP3, WfmHP4, WfmHP5, WfmHP6, WfmHP7, WfmHP8, WfmHP9, WfmHP10, WfmBathtub1, WfmBathMeas1, WfmStepResp1, WfmSRHist1, WfmSDHist1, WfmTJHist1, WfmDJHist1, WfmDDJHist1, WfmPJHist1, WfmRJOHist1, WfmSRTrack1, WfmTJTrack1, WfmDJTrack1, WfmDDJTrack1, WfmPJTrack1, WfmRJTrack1, WfmTJSpectrum1, WfmDDJSpectrum1, WfmPJSpectrum1, WfmRJSpectrum1, WfmSEye1, WfmBathtub2, WfmBathMeas2, WfmStepResp2, WfmSRHist2, WfmSDHist2, WfmTJHist2, WfmDJHist2, WfmDDJHist2, WfmPJHist2, WfmRJOHist2, WfmSRTrack2, WfmSDTrack2, WfmTJTrack2, WfmDDJTrack2, WfmPJTrack2, WfmRJTrack2, WfmTJSpectrum2, WfmDDJSpectrum2, WfmPJSpectrum2, WfmRJSpectrum2, WfmSEye2, WfmNBathtub1, WfmNBathMeas1, WfmTNHist1, WfmDNHist1, WfmDDNHist1, WfmPNHist1, WfmRNOTrack1, WfmTNTrack1, WfmDDNTrack1, WfmPNTrack1, WfmRNTrack1, WfmTNSpectrum1, WfmDDNSpectrum1, WfmPNSpectrum1, WfmRNSpectrum1, WfmNBathtub2, WfmNBathMeas2, WfmTNHist2, WfmDNHist2, WfmDDNHist2, WfmPNHist2, WfmRNOHist2, WfmTNTrack2, WfmDDNTrack2, WfmPNTrack2, WfmRNTrack2, WfmTNSpectrum2, WfmDDNSpectrum2, WfmPNSpectrum2, WfmRNSpectrum2, WfmPJDHist1, WfmBUJHist1, WfmRJHist1, WfmPJDTrack1, WfmPJDSpectrum1, WfmPJDHist2, WfmBUJHist2, WfmRJHist2, WfmPJDTrack2, WfmPJDSpectrum2, WfmPNDHist1, WfmBUNHist1, WfmRNHist1, WfmPNDTrack1, WfmPNDSpectrum1, WfmPNDHist2, WfmBUNHist2, WfmRNHist2, WfmPNDTrack2, WfmPNDSpectrum2\r\n\nRemote-control command(s):\nREFLevel<m>:USRLevel"}, {"Level"=2, "Class Only"=FALSE, "Identifier"="RSSCOPE_ATTR_REFERENCE_LEVEL_DEFINITION", "Descriptive Name"="Reference Level Definition", "Data Type"=0, "Command"="REFL{WfmSuffix}:LMOD", "Access"=2, "Range Table"="rsscope_rngAbsRel", "Read Callback"="", "Write Callback"="", "Supported Models"="", "Instrument Options"="", "Flags"=0, "Help"="Defines whether the reference is configured using absolute or relative values.\n\nAvailable Repeated Capabilities:\nWfmSuffix: WfmNone, WfmC1W1, WfmC1W2, WfmC1W3, WfmC2W1, WfmC2W2, WfmC2W3, WfmC3W1, WfmC3W2, WfmC3W3, WfmC4W1, WfmC4W2, WfmC4W3, WfmMath1, WfmMath2, WfmMath3, WfmMath4, WfmRef1, WfmRef2, WfmRef3, WfmRef4, WfmXY1, WfmXY2, WfmXY3, WfmXY4, WfmMeas1, WfmMeas2, WfmMeas3, WfmMeas4, WfmMeas5, WfmMeas6, WfmMeas7, WfmMeas8, WfmSbus1, WfmSbus2, WfmSbus3, WfmSbus4, WfmD0, WfmD1, WfmD2, WfmD3, WfmD4, WfmD5, WfmD6, WfmD7, WfmD8, WfmD9, WfmD10, WfmD11, WfmD12, WfmD13, WfmD14, WfmD15, WfmMSO1, WfmMSO2, WfmMSO3, WfmMSO4, WfmTRK1, WfmTRK2, WfmTRK3, WfmTRK4, WfmTRK5, WfmTRK6, WfmTRK7, WfmTRK8, WfmSpectrum1, WfmSpectrum2, WfmSpectrum3, WfmSpectrum4, WfmSG1TL1, WfmSG1TL2, WfmSG2TL1, WfmSG2TL2, WfmSG3TL1, WfmSG3TL2, WfmSG4TL1, WfmSG4TL2, WfmEye1, WfmEye2, WfmEye3, WfmEye4, WfmZ1V1, WfmZ1V2, WfmZ1V3, WfmZ1V4, WfmZ1I1, WfmZ1I2, WfmZ1I3, WfmZ1I4, WfmZ2V1, WfmZ2V2, WfmZ2V3, WfmZ2V4, WfmZ2I1, WfmZ2I2, WfmZ2I3, WfmZ2I4, WfmDiff1, WfmDiff2, WfmCommon1, WfmCommon2, WfmTDRZ, WfmTDRH, WfmTDRR, WfmMath5, WfmMath6, WfmMath7, WfmMath8, WfmSpectrum5, WfmSpectrum6, WfmSpectrum7, WfmSpectrum8, WfmSG5TL1, WfmSG5TL2, WfmSG6TL1, WfmSG6TL2, WfmSG7TL1, WfmSG7TL2, WfmSG8TL1, WfmSG8TL2, WfmHP1, WfmHP2, WfmHP3, WfmHP4, WfmHP5, WfmHP6, WfmHP7, WfmHP8, WfmHP9, WfmHP10, WfmBathtub1, WfmBathMeas1, WfmStepResp1, WfmSRHist1, WfmSDHist1, WfmTJHist1, WfmDJHist1, WfmDDJHist1, WfmPJHist1, WfmRJOHist1, WfmSRTrack1, WfmTJTrack1, WfmDJTrack1, WfmDDJTrack1, WfmPJTrack1, WfmRJTrack1, WfmTJSpectrum1, WfmDDJSpectrum1, WfmPJSpectrum1, WfmRJSpectrum1, WfmSEye1, WfmBathtub2, WfmBathMeas2, WfmStepResp2, WfmSRHist2, WfmSDHist2, WfmTJHist2, WfmDJHist2, WfmDDJHist2, WfmPJHist2, WfmRJOHist2, WfmSRTrack2, WfmSDTrack2, WfmTJTrack2, WfmDDJTrack2, WfmPJTrack2, WfmRJTrack2, WfmTJSpectrum2, WfmDDJSpectrum2, WfmPJSpectrum2, WfmRJSpectrum2, WfmSEye2, WfmNBathtub1, WfmNBathMeas1, WfmTNHist1, WfmDNHist1, WfmDDNHist1, WfmPNHist1, WfmRNOTrack1, WfmTNTrack1, WfmDDNTrack1, WfmPNTrack1, WfmRNTrack1, WfmTNSpectrum1, WfmDDNSpectrum1, WfmPNSpectrum1, WfmRNSpectrum1, WfmNBathtub2, WfmNBathMeas2, WfmTNHist2, WfmDNHist2, WfmDDNHist2, WfmPNHist2, WfmRNOHist2, WfmTNTrack2, WfmDDNTrack2, WfmPNTrack2, WfmRNTrack2, WfmTNSpectrum2, WfmDDNSpectrum2, WfmPNSpectrum2, WfmRNSpectrum2, WfmPJDHist1, WfmBUJHist1, WfmRJHist1, WfmPJDTrack1, WfmPJDSpectrum1, WfmPJDHist2, WfmBUJHist2, WfmRJHist2, WfmPJDTrack2, WfmPJDSpectrum2, WfmPNDHist1, WfmBUNHist1, WfmRNHist1, WfmPNDTrack1, WfmPNDSpectrum1, WfmPNDHist2, WfmBUNHist2, WfmRNHist2, WfmPNDTrack2, WfmPNDSpectrum2\r\n\nRemote-control command(s):\nREFLevel<m>:LMODe"}, {"Level"=2, "Class Only"=FALSE, "Identifier"="RSSCOPE_ATTR_REFERENCE_LEVEL_AUTO_MODE", "Descriptive Name"="Reference Level Auto Mode", "Data Type"=0, "Command"="REFL{WfmSuffix}:AUTO:MODE", "Access"=2, "Range Table"="rsscope_rngRefLevelAutoMode", "Read Callback"="", "Write Callback"="", "Supported Models"="", "Instrument Options"="", "Flags"=0, "Help"="Defines which signal level is used as a reference.\n\nAvailable Repeated Capabilities:\nWfmSuffix: WfmNone, WfmC1W1, WfmC1W2, WfmC1W3, WfmC2W1, WfmC2W2, WfmC2W3, WfmC3W1, WfmC3W2, WfmC3W3, WfmC4W1, WfmC4W2, WfmC4W3, WfmMath1, WfmMath2, WfmMath3, WfmMath4, WfmRef1, WfmRef2, WfmRef3, WfmRef4, WfmXY1, WfmXY2, WfmXY3, WfmXY4, WfmMeas1, WfmMeas2, WfmMeas3, WfmMeas4, WfmMeas5, WfmMeas6, WfmMeas7, WfmMeas8, WfmSbus1, WfmSbus2, WfmSbus3, WfmSbus4, WfmD0, WfmD1, WfmD2, WfmD3, WfmD4, WfmD5, WfmD6, WfmD7, WfmD8, WfmD9, WfmD10, WfmD11, WfmD12, WfmD13, WfmD14, WfmD15, WfmMSO1, WfmMSO2, WfmMSO3, WfmMSO4, WfmTRK1, WfmTRK2, WfmTRK3, WfmTRK4, WfmTRK5, WfmTRK6, WfmTRK7, WfmTRK8, WfmSpectrum1, WfmSpectrum2, WfmSpectrum3, WfmSpectrum4, WfmSG1TL1, WfmSG1TL2, WfmSG2TL1, WfmSG2TL2, WfmSG3TL1, WfmSG3TL2, WfmSG4TL1, WfmSG4TL2, WfmEye1, WfmEye2, WfmEye3, WfmEye4, WfmZ1V1, WfmZ1V2, WfmZ1V3, WfmZ1V4, WfmZ1I1, WfmZ1I2, WfmZ1I3, WfmZ1I4, WfmZ2V1, WfmZ2V2, WfmZ2V3, WfmZ2V4, WfmZ2I1, WfmZ2I2, WfmZ2I3, WfmZ2I4, WfmDiff1, WfmDiff2, WfmCommon1, WfmCommon2, WfmTDRZ, WfmTDRH, WfmTDRR, WfmMath5, WfmMath6, WfmMath7, WfmMath8, WfmSpectrum5, WfmSpectrum6, WfmSpectrum7, WfmSpectrum8, WfmSG5TL1, WfmSG5TL2, WfmSG6TL1, WfmSG6TL2, WfmSG7TL1, WfmSG7TL2, WfmSG8TL1, WfmSG8TL2, WfmHP1, WfmHP2, WfmHP3, WfmHP4, WfmHP5, WfmHP6, WfmHP7, WfmHP8, WfmHP9, WfmHP10, WfmBathtub1, WfmBathMeas1, WfmStepResp1, WfmSRHist1, WfmSDHist1, WfmTJHist1, WfmDJHist1, WfmDDJHist1, WfmPJHist1, WfmRJOHist1, WfmSRTrack1, WfmTJTrack1, WfmDJTrack1, WfmDDJTrack1, WfmPJTrack1, WfmRJTrack1, WfmTJSpectrum1, WfmDDJSpectrum1, WfmPJSpectrum1, WfmRJSpectrum1, WfmSEye1, WfmBathtub2, WfmBathMeas2, WfmStepResp2, WfmSRHist2, WfmSDHist2, WfmTJHist2, WfmDJHist2, WfmDDJHist2, WfmPJHist2, WfmRJOHist2, WfmSRTrack2, WfmSDTrack2, WfmTJTrack2, WfmDDJTrack2, WfmPJTrack2, WfmRJTrack2, WfmTJSpectrum2, WfmDDJSpectrum2, WfmPJSpectrum2, WfmRJSpectrum2, WfmSEye2, WfmNBathtub1, WfmNBathMeas1, WfmTNHist1, WfmDNHist1, WfmDDNHist1, WfmPNHist1, WfmRNOTrack1, WfmTNTrack1, WfmDDNTrack1, WfmPNTrack1, WfmRNTrack1, WfmTNSpectrum1, WfmDDNSpectrum1, WfmPNSpectrum1, WfmRNSpectrum1, WfmNBathtub2, WfmNBathMeas2, WfmTNHist2, WfmDNHist2, WfmDDNHist2, WfmPNHist2, 
